vi "Configure Bus Source (AUDIO - Clock).vi"(0 "VISA resource name":refnum<visa-resource-name>, 5 "BUS Number (9: Bus 1)":u16(ring)=9 items=["Bus 1"=9, "Bus 2"=10, "Bus 3"=11, "Bus 4"=12], 7 "Clock Source (0: Channel 1)":u16(ring) items=["Channel 1"=0, "Channel 2"=1, "Channel 3"=2, "Channel 4"=3, "Digital Channel 0"=14, "Digital Channel 1"=15, "Digital Channel 2"=16, "Digital Channel 3"=17, "Digital Channel 4"=18, "Digital Channel 5"=19, "Digital Channel 6"=20, "Digital Channel 7"=21, "Digital Channel 8"=22, "Digital Channel 9"=23, "Digital Channel 10"=24, "Digital Channel 11"=25, "Digital Channel 12"=26, "Digital Channel 13"=27, "Digital Channel 14"=28, "Digital Channel 15"=29], 9 "Clock Polarity (0: Fall)":u16(ring) items=["Fall", "Rise"], 11 "error in (no error)":errorcluster) -> (4 "VISA resource name out":refnum<visa-resource-name>, 15 "error out":errorcluster)   [LabVIEW 2009, in "Tektronix DPO MSO 2000 4000 Series.lvlib"]
doc: "This VI configures the clock settings for AUDIO bus.\n\n<B>Note:</B> This VI is only valid if you have installed the AUDIO application module."
uses:
  <instrlib>/Tektronix DPO MSO 2000 4000 Series/Tektronix DPO MSO 2000 4000 Series.lvlib
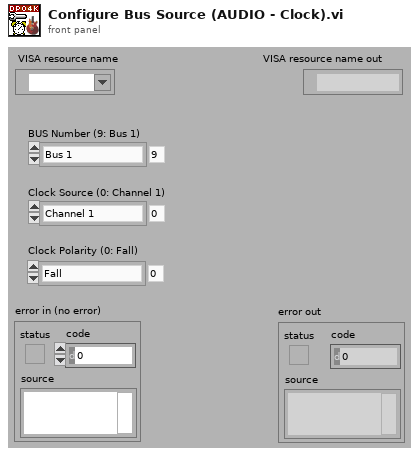
[diagram p1: front panel]
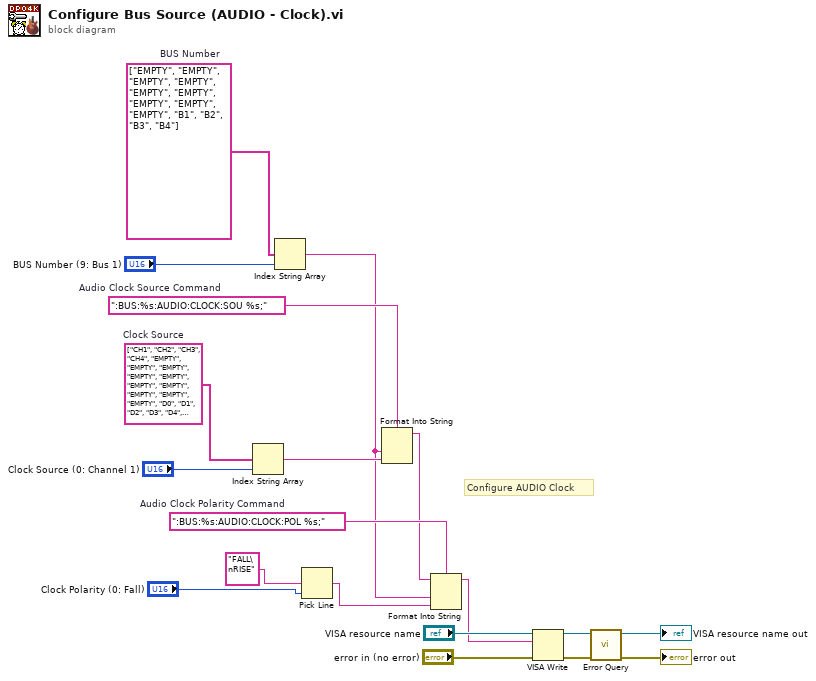
[diagram p0: block diagram]
diagram:
  w11 = ":BUS:%s:AUDIO:CLOCK:POL %s;"  # Audio Clock Polarity Command
  w16 = string[] ["CH1", "CH2", "CH3", "CH4", "EMPTY", "EMPTY", "EMPTY", "EMPTY", "EMPTY", "EMPTY", "EMPTY", "EMPTY", "EMPTY", "EMPTY", "D0", "D1", "D2", "D3", "D4", "D5", "D6", "D7", "D8", "D9", "D10", "D11", "D12", "D13", "D14", "D15"]  # Clock Source
  w17 = ":BUS:%s:AUDIO:CLOCK:SOU %s;"  # Audio Clock Source Command
  w19 = string[] ["EMPTY", "EMPTY", "EMPTY", "EMPTY", "EMPTY", "EMPTY", "EMPTY", "EMPTY", "EMPTY", "B1", "B2", "B3", "B4"]  # BUS Number
  # "Configure AUDIO Clock"
  n1 = Index String Array(1:"Clock Source (0: Channel 1)", 2:w16) -> (0:w14:string)  [unwired: 1 in]
  n2 = Index String Array(1:"BUS Number (9: Bus 1)", 2:w19) -> (0:w9:string)  [unwired: 1 in]
  n3 = Pick Line(multi-line string="FALL\nRISE", line index="Clock Polarity (0: Fall)") -> (output string=w10:string)  [unwired: 1 in]
  n4 = Format Into String(format string=w17, w9, w14) -> (resulting string=w8:string)  [unwired: 2 in, 1 out]
  n5 = Format Into String(format string=w11, initial string=w8, w9, w10) -> (resulting string=w5:string)  [unwired: 1 in, 1 out]
  n6 = VISA Write(VISA resource name="VISA resource name", write buffer=w5, error in (no error)="error in (no error)") -> (VISA resource name out=w4:refnum<visa-resource-name>, error out=w3:errorcluster)  [unwired: 1 out]
  n7 = call <instrlib>:"Error Query.vi"("error in (no error)"=w3, "VISA resource name"=w4) -> ("error out"=→"error out":errorcluster, "VISA resource name out"=→"VISA resource name out":refnum<visa-resource-name>)  [unwired: 6 in, 2 out]
